vi "errorCheck.vi"(8 "errorIn":errorcluster, 9 "from":string, 10 "errorHandler":string="Error", 11 "refer":refnum<queue>) -> (0 "errorOut":errorcluster, 3 "refer":refnum<queue>)   [LabVIEW 2017]
doc: "refer：队列索引\nerrorHandler：消息执行器中错误处理帧的名称\nfrom：检查错误发生的帧名称"
uses:
  models/EMSGData.ctl
  subvi/sendSingle.vi
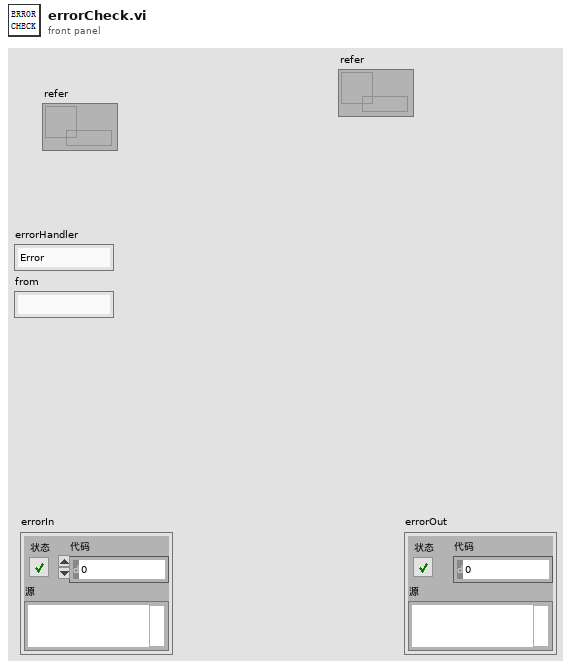
[diagram p1: front panel]
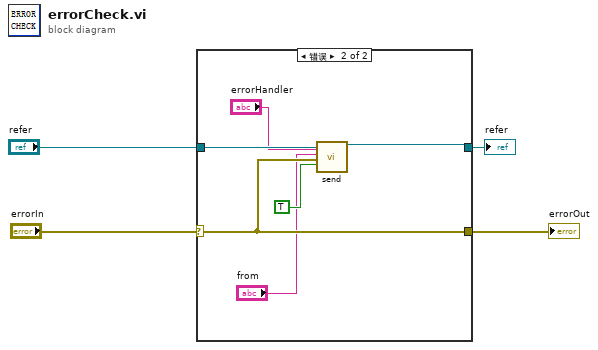
[diagram p0: block diagram]
diagram:
  n1 = case shown="错误" "errorIn" {
    selector: "errorIn" -> [w6 w8]
    tunnel: "refer" -> [w5 w12]
    tunnel: [w6 w8] -> w2
    tunnel: [w5 w11] -> w1
    frame No Error {
    }
    frame Error {
      n2 = call-poly "send.vi"("refer"=w12, "to"="errorHandler", "from"="from", "data"=w8, "priority"=TRUE) -> ("refer"=w11:refnum<queue>)  [unwired: 13 in, 1 out]
    }
  }
  "errorOut" <- w2
  "refer" <- w1
